vi "Write Elevator Position.vi"(8 "error in (no error)":errorcluster, 10 "Elevator Position":T1 scale=1.0..4.0, 11 "Sensor Interface in":refnum<class "Sensor Interface.lvclass">) -> (0 "error out":errorcluster, 3 "Sensor Interface out":refnum<class "Sensor Interface.lvclass">)   [LabVIEW 2019, in "Sensor Interface Actor.lvlib" / "Sensor Interface.lvclass"]
uses:
  Sensor Interface.lvclass
  Elevator Position.ctl
  Sensor Interface.lvclass/Sensor Interface.ctl
  Abstract Sensor Interface Actor/Abstract Sensor Interface/Abstract Sensor Interface.lvclass
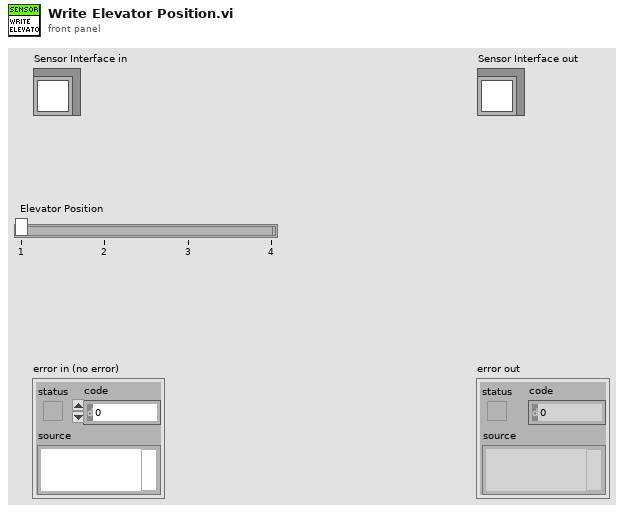
[diagram p1: front panel]
types:
  T1 = typedef "Sensor Interface Actor.lvlib/Sensor Interface.lvclass/Elevator Position.ctl" = u8
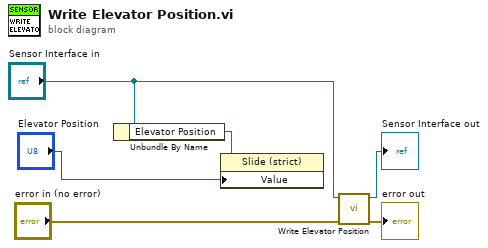
[diagram p0: block diagram]
diagram:
  n1 = Unbundle By Name("Sensor Interface in") -> ("Elevator Position"=w2:refnum<vi>)
  n2 = property class="Slide (strict)"(reference=w2, "Value"="Elevator Position") -> ()  [unwired: 1 in, 2 out]
  n3 = call-parent "Write Elevator Position.vi"("error in (no error)"="error in (no error)", "Abstract Sensor Interface in"="Sensor Interface in") -> ("error out"=→"error out":errorcluster, "Abstract Sensor Interface out"=→"Sensor Interface out":refnum<class "Sensor Interface.lvclass">)  [unwired: 8 in]
